vi "QuP Multiplexer Control.vi"() -> ()   [LabVIEW 2020, in "QuPMXdriver.lvlib"]
uses:
  QuPMXdriver.lvlib
  91754cce-ab52-4237-b78a-64c01c446f44.vi
  32ad12f4-2c8c-4504-800a-0d774754ae80.vi
  bf4f7028-8ca7-4759-aadb-7144e2be3c91.vi
  040f1b57-66c1-4072-aa26-6ea72dd8171f.vi
  6aed5eb3-691d-4dc6-b830-00691c629857.vi
  Sequence Editor.vi
  <vilib>/Comparison/Equal/Equal Functor/Equal Functor.lvclass
  cf69aa09-ab28-4be9-8615-1d2717454787.vi
panel:
  out "dummy for event \"check channels\"":bool
  in  "Set to sequence line:":i32=2 min=1 step=1
  in  "set sq line":bool
  out "Connected\nboards":bool[](array[boolean])
  in  "Get sq from MX":bool
  in  "Load sq to MX":bool
  in  "no sequences get":bool
  out "Number of sequence lines:":i32 min=0 step=1
  in  "sequence editor":bool
  out "Guards ref array":refnum<vi>[][](array[refnum])
  in  "G5C1":bool
  in  "G5C2":bool
  in  "G6C1":bool
  in  "G6C2":bool
  in  "G4C1":bool
  in  "G4C2":bool
  in  "G3C1":bool
  in  "G3C2":bool
  in  "G2C1":bool
  in  "G2C2":bool
  in  "G1C1":bool
  in  "G1C2":bool
  out "No. of connected slave boards:":u32
  out "Slaves ref array":refnum<vi>[][](array[refnum])
  in  "S5C1":bool
  in  "S5C2":bool
  in  "S6C1":bool
  in  "S6C2":bool
  in  "S4C1":bool
  in  "S4C2":bool
  in  "S3C1":bool
  in  "S3C2":bool
  in  "S2C1":bool
  in  "S2C2":bool
  in  "S1C1":bool
  in  "S1C2":bool
  in  "init":bool
  in  "Get Status":bool
  out "Ready?":bool=TRUE
  out "Enabled":bool=TRUE
  in  "check channels":bool
  in  "delay get":bool
  in  "delay set":bool
  in  "Enable\nDelay (ms)":dbl=2.0 min=0.8
  in  "timer get":bool
  in  "timer set":bool
  in  "Timer (ms)":i32=1000 min=0 step=1
  in  "Trigger polarity":enum32{"Positive", "Negative"}(radio)
  in  "Trigger source":enum32{"Internal", "External"}(radio)
  out "FP":refnum<vi>[](array[refnum])
  in  "Operation":enum32{"Remote", "Local"}(radio)=enum."Local"
  out "ID":string
  in  "reset":bool
  in  "clear":bool
  in  "stop":bool
  in  "start":bool
  in  "resume":bool
  in  "pause":bool
  in  "Stop":bool
  out "error":errorcluster
  in  "VISA":refnum<visa-resource-name>
  # "Channels"
  # "Properties"
  # "Slave boards"
  # "1       2      3      4      5      6"
  # "Channel 1"
  # "Channel 2"
  # "1       2      3      4      5      6"
  # "Guards"
  # "Channel 1"
  # "These are buttons,\nclick it!"
  # "Channel 2"
  # "Sequence"
  # "Error"
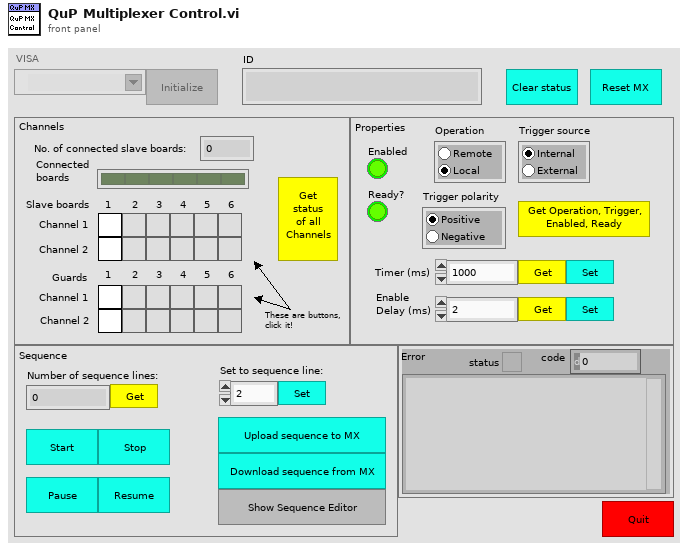
[diagram p1: front panel]
types:
  T1 = enum8{"Enabled", "Disabled", "Disabled and Grayed Out"}
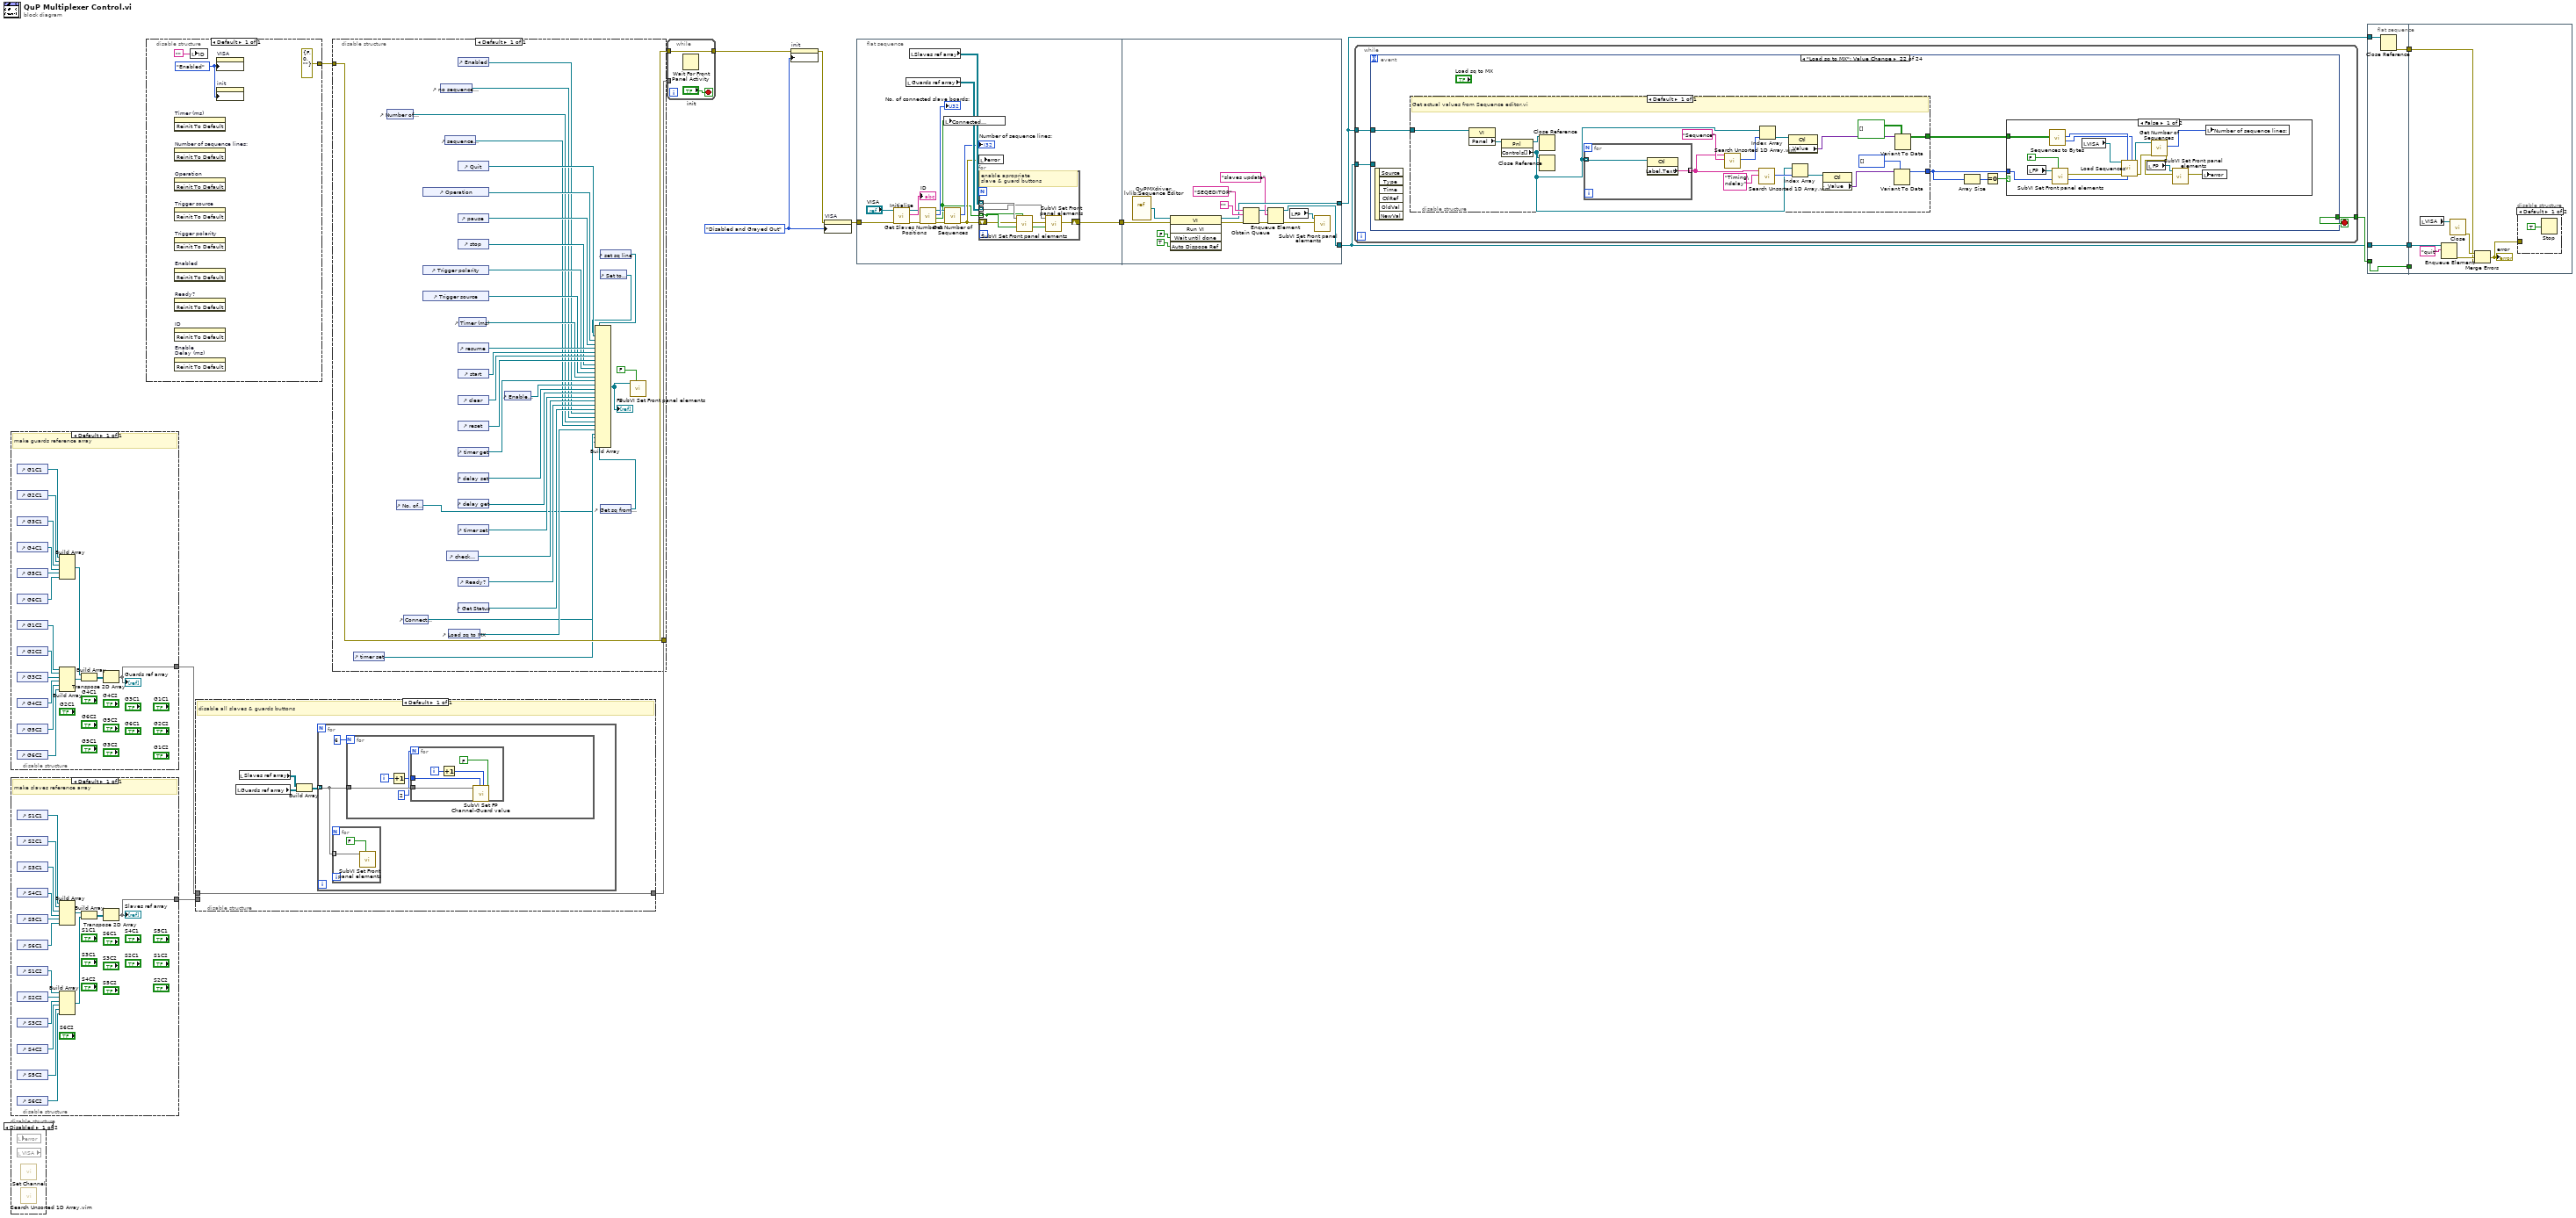
[diagram p0: block diagram]
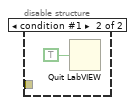
[diagram p3: hidden frame]
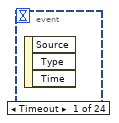
[diagram p4: hidden frame]
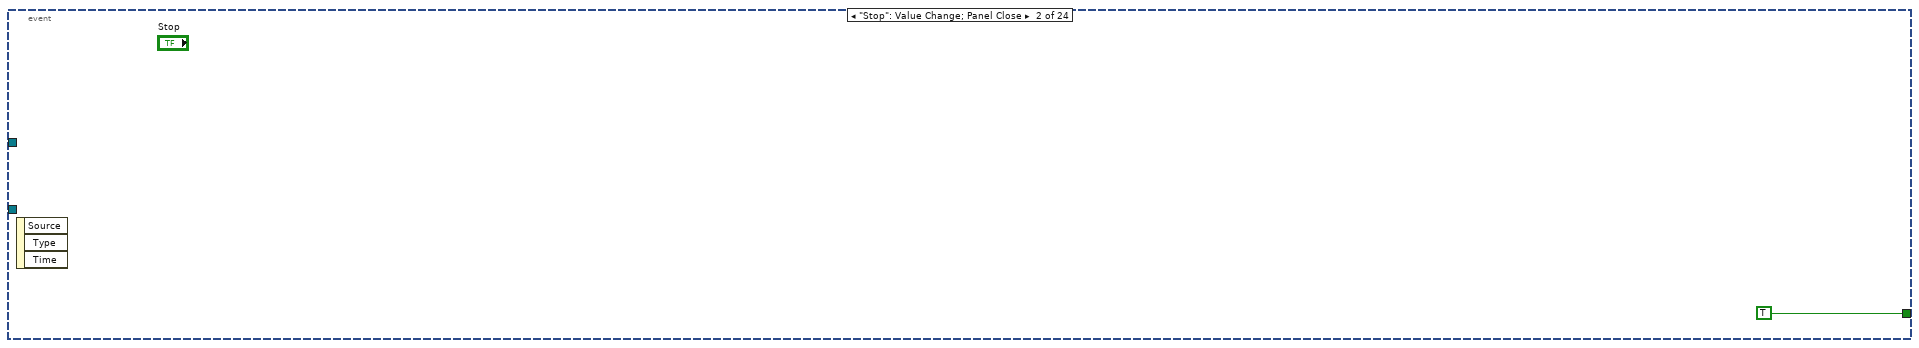
[diagram p5: hidden frame]
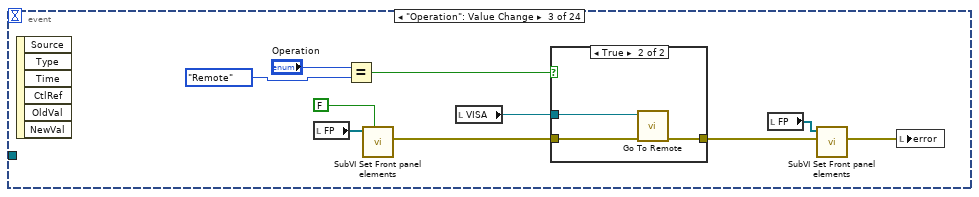
[diagram p6: hidden frame]
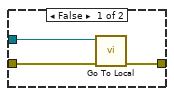
[diagram p7: hidden frame]
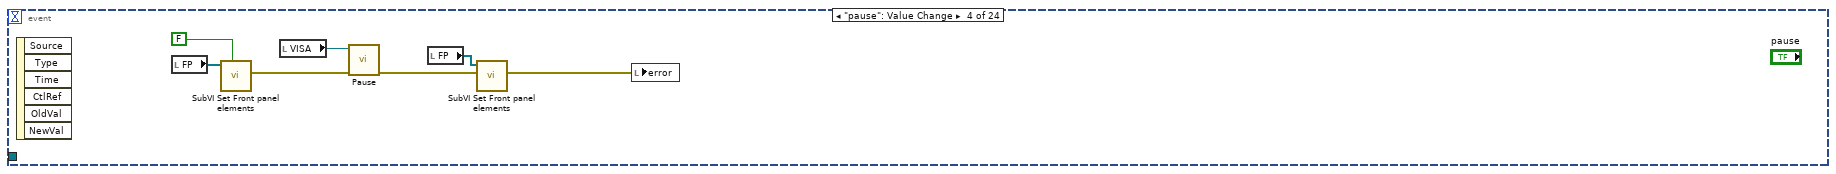
[diagram p8: hidden frame]
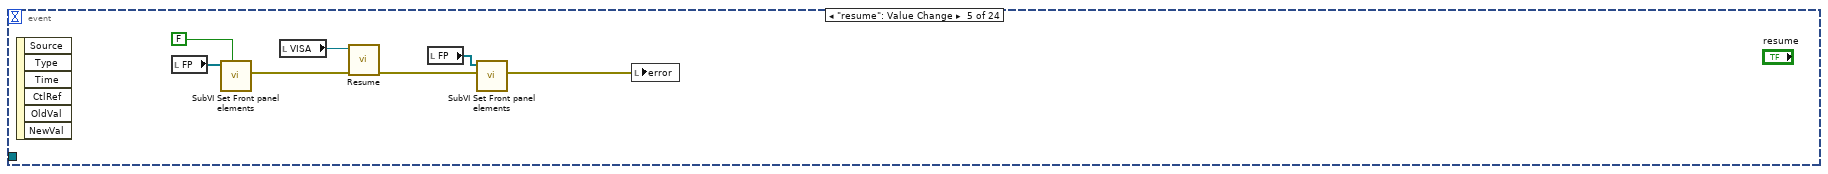
[diagram p9: hidden frame]
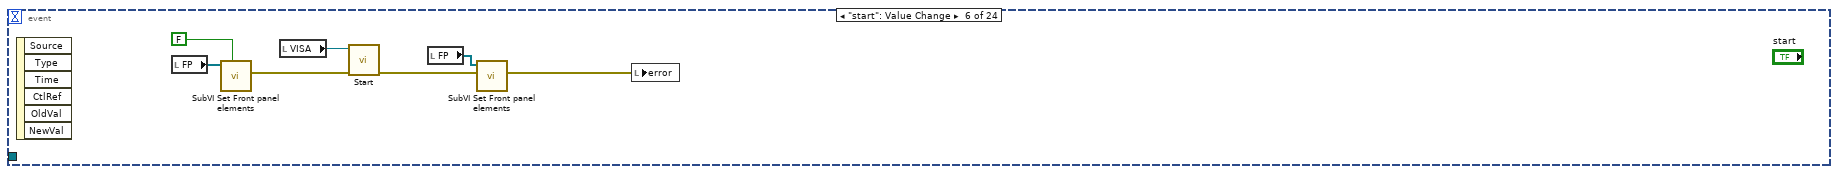
[diagram p10: hidden frame]
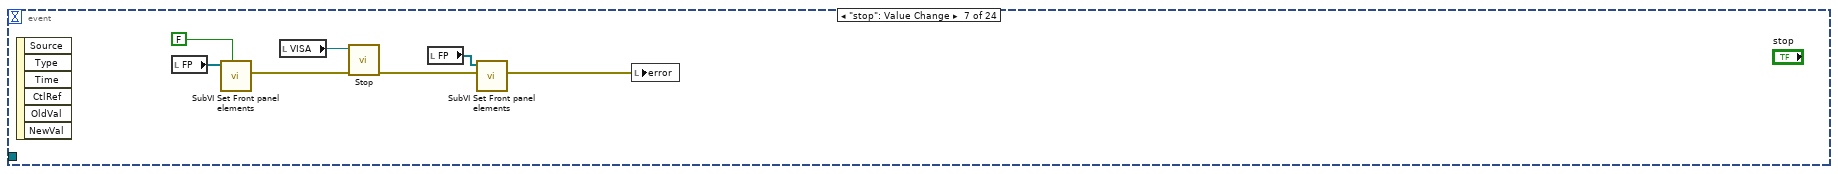
[diagram p11: hidden frame]
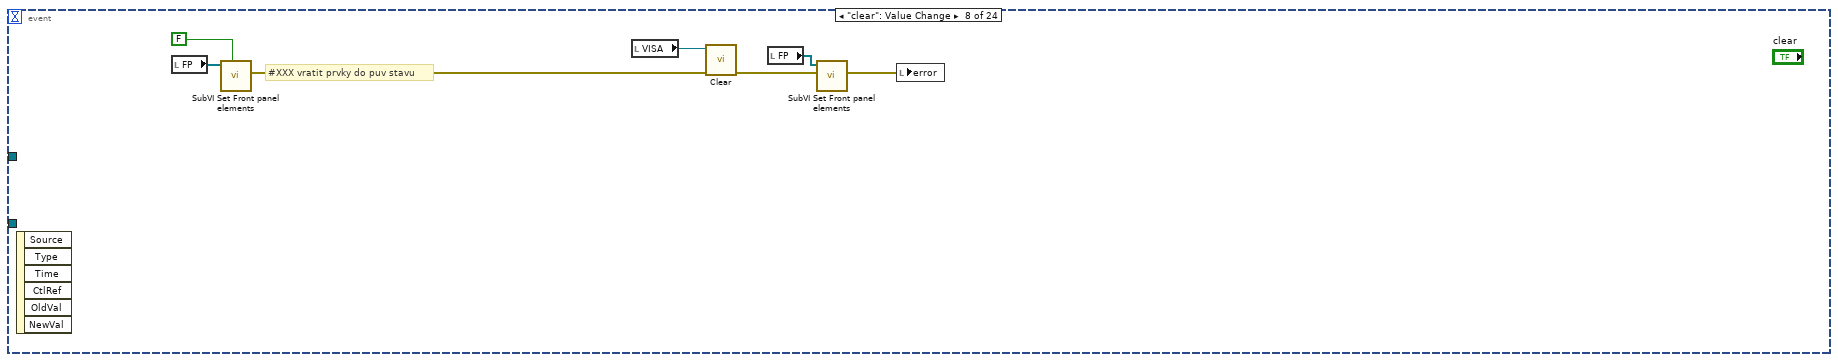
[diagram p12: hidden frame]
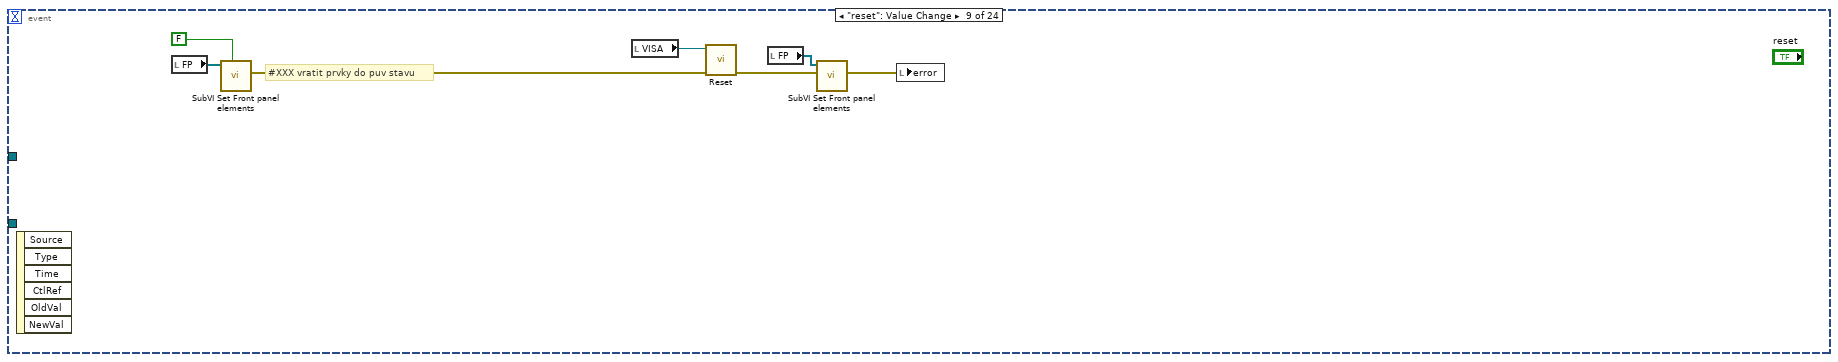
[diagram p13: hidden frame]
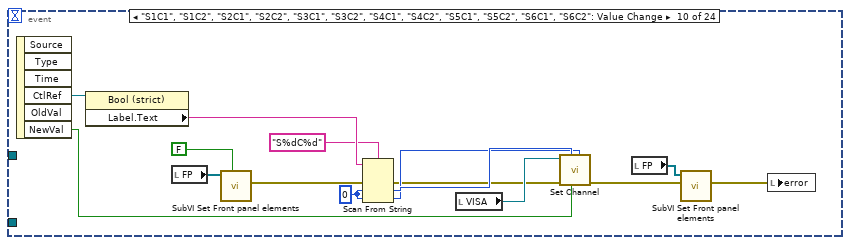
[diagram p14: hidden frame]
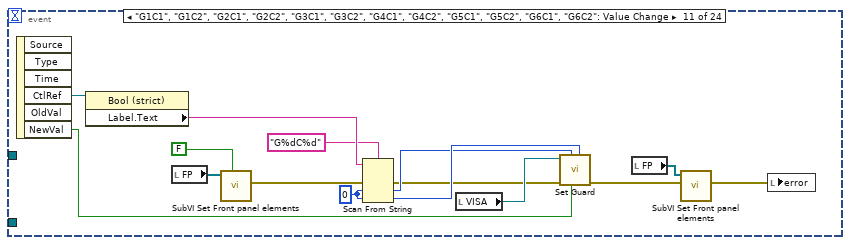
[diagram p15: hidden frame]
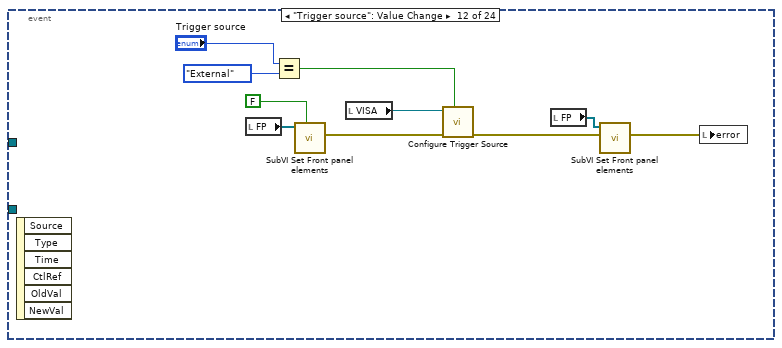
[diagram p16: hidden frame]
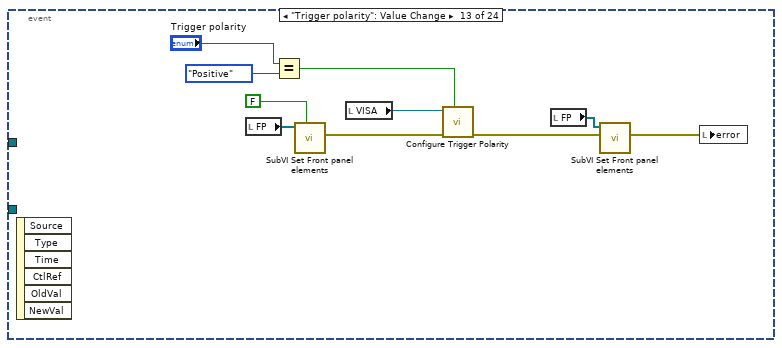
[diagram p17: hidden frame]
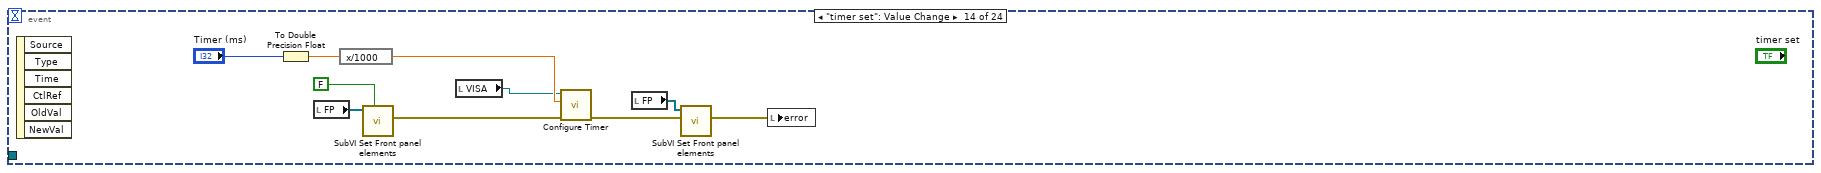
[diagram p18: hidden frame]
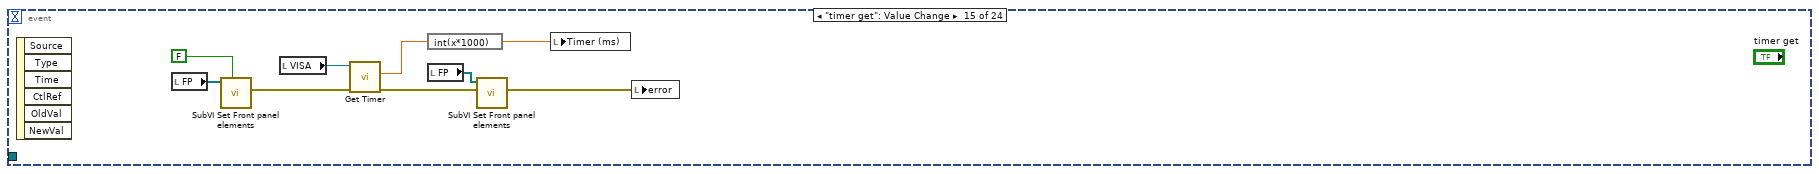
[diagram p19: hidden frame]
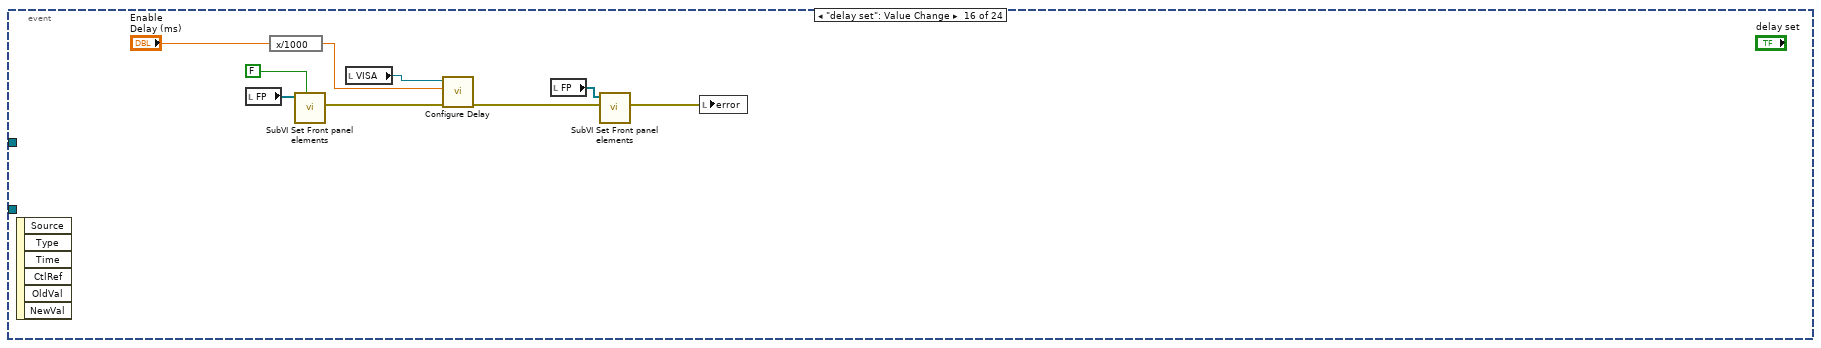
[diagram p20: hidden frame]
diagram:
  w12 = T1."Disabled and Grayed Out" ("Disabled")
  n1 = disable-structure shown="Default" {
    disable-tunnel: [w17] -> w9
    frame Enabled {
      # "make guards reference array"
      n2 = control-ref of="G1C1"() -> (w25:refnum<vi>)
      n3 = control-ref of="G2C1"() -> (w26:refnum<vi>)
      n4 = control-ref of="G3C1"() -> (w27:refnum<vi>)
      n5 = control-ref of="G4C1"() -> (w28:refnum<vi>)
      n6 = control-ref of="G5C1"() -> (w29:refnum<vi>)
      n7 = control-ref of="G6C1"() -> (w30:refnum<vi>)
      n8 = control-ref of="G1C2"() -> (w18:refnum<vi>)
      n9 = control-ref of="G2C2"() -> (w19:refnum<vi>)
      n10 = control-ref of="G3C2"() -> (w20:refnum<vi>)
      n11 = control-ref of="G4C2"() -> (w21:refnum<vi>)
      n12 = control-ref of="G5C2"() -> (w22:refnum<vi>)
      n13 = control-ref of="G6C2"() -> (w23:refnum<vi>)
      n14 = Build Array(w25, w26, w27, w28, w29, w30) -> (w24:refnum<vi>[])
      n15 = Build Array(w18, w19, w20, w21, w22, w23) -> (w31:refnum<vi>[])
      n16 = Build Array(w24, w31) -> (w32:refnum<vi>[][])
      n17 = Transpose 2D Array(2D array=w32) -> (transposed array=w17:refnum<vi>[][])
      "Guards ref array" <- w17
    }
  }
  n18 = disable-structure shown="Default" {
    disable-tunnel: [w33] -> w10
    frame Enabled {
      # "make slaves reference array"
      n19 = control-ref of="S1C1"() -> (w48:refnum<vi>)
      n20 = control-ref of="S2C1"() -> (w47:refnum<vi>)
      n21 = control-ref of="S3C1"() -> (w46:refnum<vi>)
      n22 = control-ref of="S4C1"() -> (w45:refnum<vi>)
      n23 = control-ref of="S5C1"() -> (w44:refnum<vi>)
      n24 = control-ref of="S6C1"() -> (w43:refnum<vi>)
      n25 = control-ref of="S1C2"() -> (w42:refnum<vi>)
      n26 = control-ref of="S2C2"() -> (w41:refnum<vi>)
      n27 = control-ref of="S3C2"() -> (w40:refnum<vi>)
      n28 = control-ref of="S4C2"() -> (w39:refnum<vi>)
      n29 = control-ref of="S5C2"() -> (w38:refnum<vi>)
      n30 = control-ref of="S6C2"() -> (w37:refnum<vi>)
      n31 = Build Array(w48, w47, w46, w45, w44, w43) -> (w35:refnum<vi>[])
      n32 = Build Array(w42, w41, w40, w39, w38, w37) -> (w36:refnum<vi>[])
      n33 = Build Array(w35, w36) -> (w34:refnum<vi>[][])
      n34 = Transpose 2D Array(2D array=w34) -> (transposed array=w33:refnum<vi>[][])
      "Slaves ref array" <- w33
    }
  }
  n35 = disable-structure shown="Disabled" {
    frame Disabled {
      n36 = local read "error"() -> ()  [unwired: 1 in]
      n37 = local read "VISA"() -> ()  [unwired: 1 out]
      n38 = call "Set Channel.vi"() -> ()  [unwired: 10 in, 2 out]
      n39 = call "Search Unsorted 1D Array.vim"() -> ()  [unwired: 11 in, 1 out]
    }
    frame Enabled {
    }
  }
  n40 = disable-structure shown="Default" {
    disable-tunnel: [errorcluster {"status"=FALSE, "code"=0, "source"=""} ("error in (no error)")] -> w2
    frame Enabled {
      w51 = T1."Enabled" ("Disabled")
      n41 = invoke on="Timer (ms)" class="DigNum (strict)" method="Reinit To Default"() -> ()  [unwired: 3 in, 3 out]
      n42 = invoke on="Number of sequence lines:" class="DigNum (strict)" method="Reinit To Default"() -> ()  [unwired: 3 in, 3 out]
      n43 = invoke on="Operation" class="RadioBtnsControl (strict)" method="Reinit To Default"() -> ()  [unwired: 3 in, 3 out]
      n44 = invoke on="Trigger source" class="RadioBtnsControl (strict)" method="Reinit To Default"() -> ()  [unwired: 3 in, 3 out]
      n45 = invoke on="Trigger polarity" class="RadioBtnsControl (strict)" method="Reinit To Default"() -> ()  [unwired: 3 in, 3 out]
      n46 = invoke on="Enabled" class="Bool (strict)" method="Reinit To Default"() -> ()  [unwired: 3 in, 3 out]
      n47 = invoke on="Ready?" class="Bool (strict)" method="Reinit To Default"() -> ()  [unwired: 3 in, 3 out]
      n48 = invoke on="ID" class="Str" method="Reinit To Default"() -> ()  [unwired: 3 in, 3 out]
      n49 = invoke on="Enable\nDelay (ms)" class="DigNum (strict)" method="Reinit To Default"() -> ()  [unwired: 3 in, 3 out]
      n50 = local write "ID"("") -> ()
      n51 = property on="VISA" class="VISAName"("DisabledEnum"=w51) -> ()  [unwired: 2 in, 2 out]
      n52 = property on="init" class="Bool"("DisabledEnum"=w51) -> ()  [unwired: 2 in, 2 out]
    }
  }
  n53 = disable-structure shown="Default" {
    disable-tunnel: w10 -> [_]
    disable-tunnel: w9 -> [w52]
    disable-tunnel: [w52] -> w8
    frame Enabled {
      # "disable all slaves & guards buttons"
      n54 = local read "Guards ref array"() -> (w53:refnum<vi>[][])
      n55 = local read "Slaves ref array"() -> (w55:refnum<vi>[][])
      n56 = Build Array(w55, w53) -> (w54:refnum<vi>[][][])
      n57 = for {
        tunnel: w54 -> [w56] mode=indexing
        n58 = for {
          tunnel: w56 -> [w68] mode=indexing
          n59 = call "SubVI Set Front panel elements.vi"("Enable elements (T)"=FALSE, "Array"=w68) -> ()  [unwired: 9 in, 1 out]
        }
        n60 = for {
          N: 6 -> [_]
          tunnel: w56 -> [w61]
          i -> [w59]
          n61 = Increment(x=w59) -> (x+1=w58:i32)
          n62 = for {
            N: 2 -> [_]
            tunnel: w61 -> [w66]
            tunnel: w58 -> [w64]
            i -> [w63]
            n63 = Increment(x=w63) -> (x+1=w62:i32)
            n64 = call "SubVI Set FP Channel-Guard value.vi"("Value"=FALSE, "Ch ID"=w62, "Slave ID"=w64, "Slaves ref array"=w66) -> ()  [unwired: 7 in, 1 out]
          }
        }
      }
    }
  }
  n65 = disable-structure shown="Default" {
    disable-tunnel: [w75] -> w1
    disable-tunnel: w2 -> [w75]
    frame Enabled {
      n66 = control-ref of="timer set"() -> (w74:refnum<vi>)
      n67 = control-ref of="Number of sequence lines:"() -> (w78:refnum<vi>)
      n68 = control-ref of="No. of connected slave boards:"() -> (w72:refnum<vi>)
      n69 = control-ref of="Connected\nboards"() -> (w73:refnum<vi>)
      n70 = control-ref of="Operation"() -> (w100:refnum<vi>)
      n71 = control-ref of="Trigger polarity"() -> (w91:refnum<vi>)
      n72 = control-ref of="Trigger source"() -> (w90:refnum<vi>)
      n73 = control-ref of="no sequences get"() -> (w79:refnum<vi>)
      n74 = control-ref of="sequence editor"() -> (w77:refnum<vi>)
      n75 = control-ref of="check channels"() -> (w83:refnum<vi>)
      n76 = control-ref of="Load sq to MX"() -> (w76:refnum<vi>)
      n77 = control-ref of="Enabled"() -> (w80:refnum<vi>)
      n78 = control-ref of="Quit"() -> (w101:refnum<vi>)
      n79 = control-ref of="pause"() -> (w99:refnum<vi>)
      n80 = control-ref of="stop"() -> (w92:refnum<vi>)
      n81 = control-ref of="resume"() -> (w98:refnum<vi>)
      n82 = control-ref of="start"() -> (w97:refnum<vi>)
      n83 = control-ref of="clear"() -> (w96:refnum<vi>)
      n84 = control-ref of="reset"() -> (w95:refnum<vi>)
      n85 = control-ref of="timer get"() -> (w88:refnum<vi>)
      n86 = control-ref of="delay set"() -> (w86:refnum<vi>)
      n87 = control-ref of="delay get"() -> (w85:refnum<vi>)
      n88 = control-ref of="timer set"() -> (w84:refnum<vi>)
      n89 = control-ref of="Ready?"() -> (w82:refnum<vi>)
      n90 = control-ref of="Get Status"() -> (w81:refnum<vi>)
      n91 = control-ref of="Timer (ms)"() -> (w89:refnum<vi>)
      n92 = control-ref of="Enable\nDelay (ms)"() -> (w87:refnum<vi>)
      n93 = control-ref of="set sq line"() -> (w69:refnum<vi>)
      n94 = control-ref of="Set to sequence line:"() -> (w70:refnum<vi>)
      n95 = control-ref of="Get sq from MX"() -> (w71:refnum<vi>)
      n96 = Build Array(w69, w70, w101, w100, w99, w98, w97, w96, w95, w92, w91, w90, w89, w88, w87, w86, w85, w84, w83, w82, w81, w80, w79, w78, w77, w76, w74, w73, w72, w71) -> (w94:refnum<vi>[])
      "FP" <- w94
      n97 = call "SubVI Set Front panel elements.vi"("Enable elements (T)"=FALSE ("Enable elements"), "Array"=w94) -> ()  [unwired: 9 in, 1 out]
    }
  }
  n98 = while {
    tunnel: [w102] -> w15
    tunnel: w8 -> [_]
    tunnel: w1 -> [w102]
    stop <- "init" stop-if-true
    n99 = Wait For Front Panel Activity() -> ()  [unwired: 3 in, 1 out]
  }
  n100 = property on="init" class="Bool"(error in=w15, "DisabledEnum"=w12) -> (error out=w14:errorcluster)  [unwired: 1 in, 1 out]
  n101 = property on="VISA" class="VISAName"(error in=w14, "DisabledEnum"=w12) -> (error out=w13:errorcluster)  [unwired: 1 in, 1 out]
  n102 = flat-sequence {
    tunnel: w13 -> [w117]
    tunnel: [w110] -> w11
    tunnel: w11 -> [w128]
    tunnel: [w124] -> w7
    tunnel: [w131] -> w3
    frame #0 {
      n103 = call "Initialize.vi"("error in (no error)"=w117, "VISA resource name"="VISA") -> ("error out"=w115:errorcluster, "ID"=→"ID":string, "VISA resource name out"=w114:refnum<visa-resource-name>)  [unwired: 7 in]
      n104 = local read "Guards ref array"() -> (w111:refnum<vi>[][])
      n105 = local read "Slaves ref array"() -> (w112:refnum<vi>[][])
      n106 = call "Get Slaves Number & Positions.vi"("error in (no error)"=w115, "VISA resource name"=w114) -> ("error out"=w109:errorcluster, "Connected Slaves"=w104:bool[], "No. of Slaves"=→"No. of connected slave boards:":u32, "VISA resource name out"=w107:refnum<visa-resource-name>)  [unwired: 6 in]
      n107 = local write "Connected\nboards"(w104) -> ()
      n108 = call "Get Number of Sequences.vi"("error in (no error)"=w109, "VISA resource name"=w107) -> ("error out"=w108:errorcluster, "Number of sequences"=→"Number of sequence lines:":i32)  [unwired: 7 in, 1 out]
      n109 = local write "error"(w108) -> ()
      n110 = for {
        tunnel: w112 -> [w123] mode=indexing
        tunnel: w104 -> [w121] mode=indexing
        tunnel: w111 -> [w122] mode=indexing
        shift-right: [w119] -> w110
        shift-left: w108 -> [w118]
        # "enable apropriate\nslave & guard buttons"
        n111 = call "SubVI Set Front panel elements.vi"("Enable elements (T)"=w121, "error in (passthrough)"=w118, "Array"=w123) -> ("error out"=w120:errorcluster)  [unwired: 8 in]
        n112 = call "SubVI Set Front panel elements.vi"("Enable elements (T)"=w121, "error in (passthrough)"=w120, "Array"=w122) -> ("error out"=w119:errorcluster)  [unwired: 8 in]
      }
    }
    frame #1 {
      n113 = vi-ref "QuPMXdriver.lvlib:Sequence Editor.vi"() -> (w136:refnum<vi>)
      n114 = invoke class="VI" method="Run VI"(reference=w136, error in=w128, "Wait until done"=FALSE ("Wait Until Done"), "Auto Dispose Ref"=TRUE ("Wait Until Done")) -> (reference out=w131:refnum<vi>, error out=w132:errorcluster)  [unwired: 1 in, 3 out]
      n115 = Obtain Queue(name (unnamed)="SEQEDITOR", element data type="", error in (no error)=w132) -> (queue out=w125:refnum<queue>, error out=w127:errorcluster)  [unwired: 2 in, 1 out]
      n116 = Enqueue Element(queue=w125, element="slaves update", error in (no error)=w127) -> (queue out=w124:refnum<queue>, error out=w126:errorcluster)  [unwired: 1 in, 1 out]
      n117 = local read "FP"() -> (w137:refnum<vi>[])
      n118 = call "SubVI Set Front panel elements.vi"("error in (passthrough)"=w126, "Array"=w137) -> ()  [unwired: 9 in, 1 out]
    }
  }
  n119 = while {
    tunnel: [w140] -> w16
    tunnel: w7 -> [w139]
    tunnel: w3 -> [w138]
    stop <- w140 stop-if-true
    n120 = event shown="[21] \"Load sq to MX\": Value Change" {
      selector: _ -> [_ _ _ _ _ _ _ _ _ _ _ _ _ _ _ _ _ _ _ _ _ _ _ _]
      dyn-events: _ -> [_ _ _ _ _ _ _ _ _ _ _ _ _ _ _ _ _ _ _ _ _ _ _ _]
      timeout: _ -> [_ _ _ _ _ _ _ _ _ _ _ _ _ _ _ _ _ _ _ _ _ _ _ _]
      tunnel: [_ TRUE ("Stop") _ _ _ _ _ _ _ _ _ _ _ _ _ _ _ _ _ _ _ _ _ _] -> w140
      tunnel: w139 -> [_ _ _ _ _ _ _ _ _ _ _ _ _ _ _ _ _ w289 _ _ w353 _ _ w430]
      tunnel: w138 -> [_ _ _ _ _ _ _ _ _ _ _ _ _ _ _ _ _ _ _ _ _ w358 w406 w433]
      event Timeout {
        n121 = event-data() -> ()  [unwired: 1 in, 3 out]
      }
      event "Stop": Value Change; Panel Close {
        n122 = event-data() -> ()  [unwired: 1 in, 3 out]
      }
      event "Operation": Value Change {
        n123 = event-data() -> ()  [unwired: 1 in, 6 out]
        n124 = local read "FP"() -> (w147:refnum<vi>[])
        n125 = Equal?(x="Operation", y=enum32{"Remote", "Local"}."Remote") -> (x = y?=w148:bool)
        n126 = call "SubVI Set Front panel elements.vi"("Enable elements (T)"=FALSE, "Array"=w147) -> ("error out"=w145:errorcluster)  [unwired: 9 in]
        n127 = local read "VISA"() -> (w151:refnum<visa-resource-name>)
        n128 = case shown="True" w148 {
          tunnel: [w154 w157] -> w144
          tunnel: w151 -> [w153 w156]
          tunnel: w145 -> [w152 w155]
          frame False {
            n129 = call "Go To Local.vi"("error in (no error)"=w152, "VISA resource name"=w153) -> ("error out"=w154:errorcluster)  [unwired: 8 in, 1 out]
          }
          frame True {
            n130 = call "Go To Remote.vi"("error in (no error)"=w155, "VISA resource name"=w156) -> ("error out"=w157:errorcluster)  [unwired: 8 in, 1 out]
          }
        }
        n131 = local read "FP"() -> (w142:refnum<vi>[])
        n132 = call "SubVI Set Front panel elements.vi"("error in (passthrough)"=w144, "Array"=w142) -> ("error out"=w143:errorcluster)  [unwired: 9 in]
        n133 = local write "error"(w143) -> ()
      }
      event "pause": Value Change {
        n134 = event-data() -> ()  [unwired: 1 in, 6 out]
        n135 = local read "FP"() -> (w163:refnum<vi>[])
        n136 = call "SubVI Set Front panel elements.vi"("Enable elements (T)"=FALSE, "Array"=w163) -> ("error out"=w160:errorcluster)  [unwired: 9 in]
        n137 = local read "VISA"() -> (w164:refnum<visa-resource-name>)
        n138 = call "Pause.vi"("error in (no error)"=w160, "VISA resource name"=w164) -> ("error out"=w159:errorcluster)  [unwired: 8 in, 1 out]
        n139 = local read "FP"() -> (w161:refnum<vi>[])
        n140 = call "SubVI Set Front panel elements.vi"("error in (passthrough)"=w159, "Array"=w161) -> ("error out"=w158:errorcluster)  [unwired: 9 in]
        n141 = local write "error"(w158) -> ()
      }
      event "resume": Value Change {
        n142 = event-data() -> ()  [unwired: 1 in, 6 out]
        n143 = local read "FP"() -> (w169:refnum<vi>[])
        n144 = call "SubVI Set Front panel elements.vi"("Enable elements (T)"=FALSE, "Array"=w169) -> ("error out"=w167:errorcluster)  [unwired: 9 in]
        n145 = local read "VISA"() -> (w171:refnum<visa-resource-name>)
        n146 = call "Resume.vi"("error in (no error)"=w167, "VISA resource name"=w171) -> ("error out"=w166:errorcluster)  [unwired: 8 in, 1 out]
        n147 = local read "FP"() -> (w170:refnum<vi>[])
        n148 = call "SubVI Set Front panel elements.vi"("error in (passthrough)"=w166, "Array"=w170) -> ("error out"=w165:errorcluster)  [unwired: 9 in]
        n149 = local write "error"(w165) -> ()
      }
      event "start": Value Change {
        n150 = event-data() -> ()  [unwired: 1 in, 6 out]
        n151 = local read "FP"() -> (w176:refnum<vi>[])
        n152 = call "SubVI Set Front panel elements.vi"("Enable elements (T)"=FALSE, "Array"=w176) -> ("error out"=w174:errorcluster)  [unwired: 9 in]
        n153 = local read "VISA"() -> (w178:refnum<visa-resource-name>)
        n154 = call "Start.vi"("error in (no error)"=w174, "VISA resource name"=w178) -> ("error out"=w173:errorcluster)  [unwired: 8 in, 1 out]
        n155 = local read "FP"() -> (w177:refnum<vi>[])
        n156 = call "SubVI Set Front panel elements.vi"("error in (passthrough)"=w173, "Array"=w177) -> ("error out"=w172:errorcluster)  [unwired: 9 in]
        n157 = local write "error"(w172) -> ()
      }
      event "stop": Value Change {
        n158 = event-data() -> ()  [unwired: 1 in, 6 out]
        n159 = local read "FP"() -> (w183:refnum<vi>[])
        n160 = call "SubVI Set Front panel elements.vi"("Enable elements (T)"=FALSE, "Array"=w183) -> ("error out"=w181:errorcluster)  [unwired: 9 in]
        n161 = local read "VISA"() -> (w185:refnum<visa-resource-name>)
        n162 = call "Stop.vi"("error in (no error)"=w181, "VISA resource name"=w185) -> ("error out"=w180:errorcluster)  [unwired: 8 in, 1 out]
        n163 = local read "FP"() -> (w184:refnum<vi>[])
        n164 = call "SubVI Set Front panel elements.vi"("error in (passthrough)"=w180, "Array"=w184) -> ("error out"=w179:errorcluster)  [unwired: 9 in]
        n165 = local write "error"(w179) -> ()
      }
      event "clear": Value Change {
        # "#XXX vratit prvky do puv stavu"
        n166 = event-data() -> ()  [unwired: 1 in, 6 out]
        n167 = local read "FP"() -> (w190:refnum<vi>[])
        n168 = call "SubVI Set Front panel elements.vi"("Enable elements (T)"=FALSE, "Array"=w190) -> ("error out"=w188:errorcluster)  [unwired: 9 in]
        n169 = local read "VISA"() -> (w192:refnum<visa-resource-name>)
        n170 = call "Clear.vi"("error in (no error)"=w188, "VISA resource name"=w192) -> ("error out"=w187:errorcluster)  [unwired: 8 in, 1 out]
        n171 = local read "FP"() -> (w191:refnum<vi>[])
        n172 = call "SubVI Set Front panel elements.vi"("error in (passthrough)"=w187, "Array"=w191) -> ("error out"=w186:errorcluster)  [unwired: 9 in]
        n173 = local write "error"(w186) -> ()
      }
      event "reset": Value Change {
        # "#XXX vratit prvky do puv stavu"
        n174 = event-data() -> ()  [unwired: 1 in, 6 out]
        n175 = local read "FP"() -> (w197:refnum<vi>[])
        n176 = call "SubVI Set Front panel elements.vi"("Enable elements (T)"=FALSE, "Array"=w197) -> ("error out"=w195:errorcluster)  [unwired: 9 in]
        n177 = local read "VISA"() -> (w199:refnum<visa-resource-name>)
        n178 = call "Reset.vi"("error in (no error)"=w195, "VISA resource name"=w199) -> ("error out"=w194:errorcluster)  [unwired: 8 in, 1 out]
        n179 = local read "FP"() -> (w198:refnum<vi>[])
        n180 = call "SubVI Set Front panel elements.vi"("error in (passthrough)"=w194, "Array"=w198) -> ("error out"=w193:errorcluster)  [unwired: 9 in]
        n181 = local write "error"(w193) -> ()
      }
      event "S1C1", "S1C2", "S2C1", "S2C2", "S3C1", "S3C2", "S4C1", "S4C2", "S5C1", "S5C2", "S6C1", "S6C2": Value Change {
        w200 = 0 ("default value 1")
        n182 = event-data() -> ("CtlRef"=w214:refnum<vi>, "NewVal"=w208:bool)  [unwired: 1 in, 4 out]
        n183 = property class="Bool (strict)"(reference=w214) -> ("Label.Text"=w213:string)  [unwired: 1 in, 2 out]
        n184 = local read "FP"() -> (w203:refnum<vi>[])
        n185 = call "SubVI Set Front panel elements.vi"("Enable elements (T)"=FALSE, "Array"=w203) -> ("error out"=w201:errorcluster)  [unwired: 9 in]
        n186 = Scan From String(format string="S%dC%d", input string=w213, error in=w201, default 1=w200, default 2=w200) -> (error out=w207:errorcluster, output 1=w211:i32, output 2=w210:i32)  [unwired: 1 in, 2 out]
        n187 = local read "VISA"() -> (w209:refnum<visa-resource-name>)
        n188 = call "Set Channel.vi"("Channel"=w210, "Channel Status"=w208, "Slave"=w211, "error in (no error)"=w207, "VISA resource name"=w209) -> ("error out"=w205:errorcluster)  [unwired: 5 in, 1 out]
        n189 = local read "FP"() -> (w206:refnum<vi>[])
        n190 = call "SubVI Set Front panel elements.vi"("error in (passthrough)"=w205, "Array"=w206) -> ("error out"=w204:errorcluster)  [unwired: 9 in]
        n191 = local write "error"(w204) -> ()
      }
      event "G1C1", "G1C2", "G2C1", "G2C2", "G3C1", "G3C2", "G4C1", "G4C2", "G5C1", "G5C2", "G6C1", "G6C2": Value Change {
        w221 = 0 ("default value 1")
        n192 = event-data() -> ("CtlRef"=w227:refnum<vi>, "NewVal"=w223:bool)  [unwired: 1 in, 4 out]
        n193 = property class="Bool (strict)"(reference=w227) -> ("Label.Text"=w229:string)  [unwired: 1 in, 2 out]
        n194 = local read "FP"() -> (w220:refnum<vi>[])
        n195 = call "SubVI Set Front panel elements.vi"("Enable elements (T)"=FALSE, "Array"=w220) -> ("error out"=w218:errorcluster)  [unwired: 9 in]
        n196 = Scan From String(format string="G%dC%d", input string=w229, error in=w218, default 1=w221, default 2=w221) -> (error out=w222:errorcluster, output 1=w225:i32, output 2=w226:i32)  [unwired: 1 in, 2 out]
        n197 = local read "VISA"() -> (w224:refnum<visa-resource-name>)
        n198 = call "Set Guard.vi"("Channel"=w226, "Channel Guard Status"=w223, "Slave"=w225, "error in (no error)"=w222, "VISA resource name"=w224) -> ("error out"=w216:errorcluster)  [unwired: 5 in, 1 out]
        n199 = local read "FP"() -> (w217:refnum<vi>[])
        n200 = call "SubVI Set Front panel elements.vi"("error in (passthrough)"=w216, "Array"=w217) -> ("error out"=w215:errorcluster)  [unwired: 9 in]
        n201 = local write "error"(w215) -> ()
      }
      event "Trigger source": Value Change {
        n202 = event-data() -> ()  [unwired: 1 in, 6 out]
        n203 = local read "FP"() -> (w237:refnum<vi>[])
        n204 = Equal?(x="Trigger source", y=enum32{"Internal", "External"}."External") -> (x = y?=w231:bool)
        n205 = call "SubVI Set Front panel elements.vi"("Enable elements (T)"=FALSE, "Array"=w237) -> ("error out"=w233:errorcluster)  [unwired: 9 in]
        n206 = local read "VISA"() -> (w235:refnum<visa-resource-name>)
        n207 = call "Configure Trigger Source.vi"("Trigger External (T)"=w231, "error in (no error)"=w233, "VISA resource name"=w235) -> ("error out"=w234:errorcluster)  [unwired: 7 in, 1 out]
        n208 = local read "FP"() -> (w238:refnum<vi>[])
        n209 = call "SubVI Set Front panel elements.vi"("error in (passthrough)"=w234, "Array"=w238) -> ("error out"=w239:errorcluster)  [unwired: 9 in]
        n210 = local write "error"(w239) -> ()
      }
      event "Trigger polarity": Value Change {
        n211 = event-data() -> ()  [unwired: 1 in, 6 out]
        n212 = local read "FP"() -> (w247:refnum<vi>[])
        n213 = Equal?(x="Trigger polarity", y=enum32{"Positive", "Negative"}."Positive") -> (x = y?=w241:bool)
        n214 = call "SubVI Set Front panel elements.vi"("Enable elements (T)"=FALSE, "Array"=w247) -> ("error out"=w245:errorcluster)  [unwired: 9 in]
        n215 = local read "VISA"() -> (w240:refnum<visa-resource-name>)
        n216 = call "Configure Trigger Polarity.vi"("Trigger Polarity Positive (T)"=w241, "error in (no error)"=w245, "VISA resource name"=w240) -> ("error out"=w244:errorcluster)  [unwired: 7 in, 1 out]
        n217 = local read "FP"() -> (w248:refnum<vi>[])
        n218 = call "SubVI Set Front panel elements.vi"("error in (passthrough)"=w244, "Array"=w248) -> ("error out"=w249:errorcluster)  [unwired: 9 in]
        n219 = local write "error"(w249) -> ()
      }
      event "timer set": Value Change {
        n220 = event-data() -> ()  [unwired: 1 in, 6 out]
        n221 = To Double Precision Float(number="Timer (ms)") -> (double precision float=w254:dbl)
        n222 = local read "FP"() -> (w257:refnum<vi>[])
        n223 = expression code="x/1000"(w254) -> (w253:dbl)
        n224 = call "SubVI Set Front panel elements.vi"("Enable elements (T)"=FALSE, "Array"=w257) -> ("error out"=w251:errorcluster)  [unwired: 9 in]
        n225 = local read "VISA"() -> (w252:refnum<visa-resource-name>)
        n226 = call "Configure Timer.vi"("error in (no error)"=w251, "Internal timer (2 s)"=w253, "VISA resource name"=w252) -> ("error out"=w250:errorcluster)  [unwired: 7 in, 1 out]
        n227 = local read "FP"() -> (w258:refnum<vi>[])
        n228 = call "SubVI Set Front panel elements.vi"("error in (passthrough)"=w250, "Array"=w258) -> ("error out"=w259:errorcluster)  [unwired: 9 in]
        n229 = local write "error"(w259) -> ()
      }
      event "timer get": Value Change {
        n230 = event-data() -> ()  [unwired: 1 in, 6 out]
        n231 = local read "FP"() -> (w266:refnum<vi>[])
        n232 = call "SubVI Set Front panel elements.vi"("Enable elements (T)"=FALSE, "Array"=w266) -> ("error out"=w264:errorcluster)  [unwired: 9 in]
        n233 = local read "VISA"() -> (w262:refnum<visa-resource-name>)
        n234 = call "Get Timer.vi"("error in (no error)"=w264, "VISA resource name"=w262) -> ("error out"=w263:errorcluster, "Internal Timer value (s)"=w261:dbl)  [unwired: 7 in, 1 out]
        n235 = expression code="int(x*1000)"(w261) -> (w260:dbl)
        n236 = local read "FP"() -> (w267:refnum<vi>[])
        n237 = call "SubVI Set Front panel elements.vi"("error in (passthrough)"=w263, "Array"=w267) -> ("error out"=w268:errorcluster)  [unwired: 9 in]
        n238 = local write "Timer (ms)"(w260) -> ()
        n239 = local write "error"(w268) -> ()
      }
      event "delay set": Value Change {
        n240 = event-data() -> ()  [unwired: 1 in, 6 out]
        n241 = local read "FP"() -> (w275:refnum<vi>[])
        n242 = expression code="x/1000"("Enable\nDelay (ms)") -> (w270:dbl)
        n243 = call "SubVI Set Front panel elements.vi"("Enable elements (T)"=FALSE, "Array"=w275) -> ("error out"=w272:errorcluster)  [unwired: 9 in]
        n244 = local read "VISA"() -> (w273:refnum<visa-resource-name>)
        n245 = call "Configure Delay.vi"("error in (no error)"=w272, "Delay (s)"=w270, "VISA resource name"=w273) -> ("error out"=w271:errorcluster)  [unwired: 7 in, 1 out]
        n246 = local read "FP"() -> (w276:refnum<vi>[])
        n247 = call "SubVI Set Front panel elements.vi"("error in (passthrough)"=w271, "Array"=w276) -> ("error out"=w277:errorcluster)  [unwired: 9 in]
        n248 = local write "error"(w277) -> ()
      }
      event "delay get": Value Change {
        n249 = event-data() -> ()  [unwired: 1 in, 6 out]
        n250 = local read "FP"() -> (w284:refnum<vi>[])
        n251 = call "SubVI Set Front panel elements.vi"("Enable elements (T)"=FALSE, "Array"=w284) -> ("error out"=w282:errorcluster)  [unwired: 9 in]
        n252 = local read "VISA"() -> (w280:refnum<visa-resource-name>)
        n253 = call "Get Delay.vi"("error in (no error)"=w282, "VISA resource name"=w280) -> ("error out"=w281:errorcluster, "Delay (s)"=w279:dbl)  [unwired: 7 in, 1 out]
        n254 = expression code="int(x*1000)"(w279) -> (w278:dbl)
        n255 = local read "FP"() -> (w285:refnum<vi>[])
        n256 = call "SubVI Set Front panel elements.vi"("error in (passthrough)"=w281, "Array"=w285) -> ("error out"=w286:errorcluster)  [unwired: 9 in]
        n257 = local write "Enable\nDelay (ms)"(w278) -> ()
        n258 = local write "error"(w286) -> ()
      }
      event "check channels", "dummy for event \"check channels\"": Value Change {
        # "this is only to get possibility\nto start this event case\neven if button \"check channels\"\nis latching"
        n259 = event-data() -> ()  [unwired: 1 in, 6 out]
        n260 = local read "FP"() -> (w301:refnum<vi>[])
        n261 = call "SubVI Set Front panel elements.vi"("Enable elements (T)"=FALSE, "Array"=w301) -> ("error out"=w294:errorcluster)  [unwired: 9 in]
        n262 = local read "VISA"() -> (w295:refnum<visa-resource-name>)
        n263 = local read "Guards ref array"() -> (w291:refnum<vi>[][])
        n264 = local read "Slaves ref array"() -> (w297:refnum<vi>[][])
        n265 = call "Get Slaves Number & Positions.vi"("error in (no error)"=w294, "VISA resource name"=w295) -> ("error out"=w292:errorcluster, "Connected Slaves"=w296:bool[], "No. of Slaves"=w298:u32)  [unwired: 6 in, 1 out]
        "Connected\nboards" <- w296
        n266 = local write "No. of connected slave boards:"(w298) -> ()
        n267 = for {
          tunnel: w297 -> [w309] mode=indexing
          tunnel: w296 -> [w305] mode=indexing
          shift-right: [w306] -> w293
          shift-left: w292 -> [w308]
          tunnel: w291 -> [w304] mode=indexing
          n268 = call "SubVI Set Front panel elements.vi"("Enable elements (T)"=w305, "error in (passthrough)"=w308, "Array"=w309) -> ("error out"=w307:errorcluster)  [unwired: 8 in]
          n269 = call "SubVI Set Front panel elements.vi"("Enable elements (T)"=w305, "error in (passthrough)"=w307, "Array"=w304) -> ("error out"=w306:errorcluster)  [unwired: 8 in]
        }
        n270 = for {
          N: 2 -> [_]
          shift-right: [w313] -> w288
          shift-left: w293 -> [w312]
          i -> [w311]
          n271 = Increment(x=w311) -> (x+1=w310:i32)
          n272 = for {
            N: 6 -> [_]
            shift-right: [w322] -> w313
            shift-left: w312 -> [w321]
            tunnel: w310 -> [w316]
            i -> [w319]
            # "#XXX no way how to check guard status?"
            n273 = local read "VISA"() -> (w320:refnum<visa-resource-name>)
            n274 = Increment(x=w319) -> (x+1=w317:i32)
            n275 = call "Get Channel Status.vi"("Channel"=w316, "Slave"=w317, "error in (no error)"=w321, "VISA resource name"=w320) -> ("error out"=w322:errorcluster, "Channel Enabled"=w315:bool)  [unwired: 5 in, 1 out]
            n276 = local read "Slaves ref array"() -> (w318:refnum<vi>[][])
            n277 = call "SubVI Set FP Channel-Guard value.vi"("Value"=w315, "Ch ID"=w316, "Slave ID"=w317, "Slaves ref array"=w318) -> ()  [unwired: 7 in, 1 out]
          }
        }
        n278 = Enqueue Element(queue=w289, element="slaves update", error in (no error)=w288) -> (error out=w287:errorcluster)  [unwired: 1 in, 2 out]
        n279 = local read "FP"() -> (w302:refnum<vi>[])
        n280 = call "SubVI Set Front panel elements.vi"("error in (passthrough)"=w287, "Array"=w302) -> ("error out"=w303:errorcluster)  [unwired: 9 in]
        n281 = local write "error"(w303) -> ()
      }
      event "Get Status": Value Change {
        n282 = event-data() -> ()  [unwired: 1 in, 6 out]
        n283 = local read "FP"() -> (w341:refnum<vi>[])
        n284 = call "SubVI Set Front panel elements.vi"("Enable elements (T)"=FALSE, "Array"=w341) -> ("error out"=w336:errorcluster)  [unwired: 9 in]
        n285 = local read "VISA"() -> (w337:refnum<visa-resource-name>)
        n286 = call "Get MX Status.vi"("error in (no error)"=w336, "VISA resource name"=w337) -> ("error out"=w335:errorcluster, "Ready?"=→"Ready?":bool, "Enabled"=→"Enabled":bool, "TRG Polarity Positive"=w330:bool, "Local?"=w334:bool, "TRG External"=w326:bool)  [unwired: 3 in, 1 out]
        n287 = local read "FP"() -> (w342:refnum<vi>[])
        n288 = Select(t=enum32{"Remote", "Local"}."Local" ("Operation"), s=w334, f=enum32{"Remote", "Local"}."Remote" ("Operation")) -> (s? t:f=w331:enum32{"Remote", "Local"})
        n289 = Select(t=enum32{"Positive", "Negative"}."Positive" ("Trigger polarity"), s=w330, f=enum32{"Positive", "Negative"}."Negative" ("Trigger polarity")) -> (s? t:f=w327:enum32{"Positive", "Negative"})
        n290 = Select(t=enum32{"Internal", "External"}."External" ("Trigger source"), s=w326, f=enum32{"Internal", "External"}."Internal" ("Trigger source")) -> (s? t:f=w323:enum32{"Internal", "External"})
        n291 = call "SubVI Set Front panel elements.vi"("error in (passthrough)"=w335, "Array"=w342) -> ("error out"=w343:errorcluster)  [unwired: 9 in]
        n292 = local write "Operation"(w331) -> ()
        n293 = local write "Trigger polarity"(w327) -> ()
        n294 = local write "Trigger source"(w323) -> ()
        n295 = local write "error"(w343) -> ()
      }
      event "no sequences get": Value Change {
        n296 = event-data() -> ()  [unwired: 1 in, 6 out]
        n297 = local read "FP"() -> (w349:refnum<vi>[])
        n298 = call "SubVI Set Front panel elements.vi"("Enable elements (T)"=FALSE, "Array"=w349) -> ("error out"=w347:errorcluster)  [unwired: 9 in]
        n299 = local read "VISA"() -> (w345:refnum<visa-resource-name>)
        n300 = call "Get Number of Sequences.vi"("error in (no error)"=w347, "VISA resource name"=w345) -> ("error out"=w346:errorcluster, "Number of sequences"=w344:i32)  [unwired: 7 in, 1 out]
        n301 = local read "FP"() -> (w350:refnum<vi>[])
        n302 = local write "Number of sequence lines:"(w344) -> ()
        n303 = call "SubVI Set Front panel elements.vi"("error in (passthrough)"=w346, "Array"=w350) -> ("error out"=w351:errorcluster)  [unwired: 9 in]
        n304 = local write "error"(w351) -> ()
      }
      event "sequence editor": Value Change {
        n305 = event-data() -> ()  [unwired: 1 in, 6 out]
        n306 = Enqueue Element(queue=w353, element="FP open") -> ()  [unwired: 2 in, 3 out]
      }
      event "Load sq to MX": Value Change {
        n307 = event-data() -> ()  [unwired: 1 in, 6 out]
        n308 = disable-structure shown="Default" {
          disable-tunnel: w358 -> [w390]
          disable-tunnel: [w375] -> w357
          disable-tunnel: [w374] -> w356
          frame Enabled {
            # "Get actual values from Sequence editor.vi"
            n309 = property class="VI"(reference=w390) -> ("Panel"=w389:refnum<vi>)  [unwired: 1 in, 2 out]
            n310 = property class="Pnl"(reference=w389) -> (reference out=w376:refnum<vi>, "Controls[]"=w377:refnum<vi>[])  [unwired: 1 in, 1 out]
            n311 = Close Reference(reference=w376) -> ()  [unwired: 1 in, 1 out]
            n312 = Close Reference(reference=w377) -> ()  [unwired: 1 in, 1 out]
            n313 = for {
              tunnel: w377 -> [w392] mode=indexing
              tunnel: [w391] -> w379 mode=indexing
              n314 = property class="Ctl"(reference=w392) -> ("Label.Text"=w391:string)  [unwired: 1 in, 2 out]
            }
            n315 = call "Search Unsorted 1D Array.vim"("element"="Sequence" ("Label.Text"), "unsorted 1D array"=w379) -> ("index of element"=w381:i32)  [unwired: 9 in]
            n316 = call "Search Unsorted 1D Array.vim"("element"="Timing\ndelay" ("Label.Text"), "unsorted 1D array"=w379) -> ("index of element"=w387:i32)  [unwired: 9 in]
            n317 = Index Array(array=w377, index=w381) -> (element=w382:refnum<vi>)
            n318 = property class="Ctl"(reference=w382) -> ("Value"=w383:variant)  [unwired: 1 in, 2 out]
            n319 = Index Array(array=w377, index=w387) -> (element=w386:refnum<vi>)
            n320 = property class="Ctl"(reference=w386) -> ("Value"=w385:variant)  [unwired: 1 in, 2 out]
            n321 = Variant To Data(type=u8[] [] ("Ch. bytes 2"), Variant=w385) -> (data=w374:u8[])  [unwired: 1 in, 1 out]
            n322 = Variant To Data(type=bool[][] [], Variant=w383) -> (data=w375:bool[][])  [unwired: 1 in, 1 out]
          }
        }
        n323 = Array Size(array=w356) -> (size(s)=w355:i32)
        n324 = Equal To 0?(x=w355) -> (x = 0?=w354:bool)
        n325 = case shown="False" w354 {
          tunnel: w357 -> [w364 _]
          tunnel: w356 -> [w363 _]
          frame False {
            n326 = local read "FP"() -> (w368:refnum<vi>[])
            n327 = call "Sequences to Bytes.vi"("Channel states"=w364) -> ("Ch. bytes 2"=w371:u8[], "Ch. bytes 1"=w372:u8[])  [unwired: 9 in]
            n328 = call "SubVI Set Front panel elements.vi"("Enable elements (T)"=FALSE, "Array"=w368) -> ("error out"=w366:errorcluster)  [unwired: 9 in]
            n329 = local read "VISA"() -> (w365:refnum<visa-resource-name>)
            n330 = call "Load Sequences.vi"("Byte 2 Ch."=w371, "Byte 3 Timing Delay"=w363, "Byte 1 Ch."=w372, "error in (no error)"=w366, "VISA resource name"=w365) -> ("error out"=w361:errorcluster, "VISA resource name out"=w359:refnum<visa-resource-name>)  [unwired: 5 in]
            n331 = local read "FP"() -> (w369:refnum<vi>[])
            n332 = call "Get Number of Sequences.vi"("error in (no error)"=w361, "VISA resource name"=w359) -> ("error out"=w360:errorcluster, "Number of sequences"=w362:i32)  [unwired: 7 in, 1 out]
            n333 = call "SubVI Set Front panel elements.vi"("error in (passthrough)"=w360, "Array"=w369) -> ("error out"=w370:errorcluster)  [unwired: 9 in]
            n334 = local write "error"(w370) -> ()
            n335 = local write "Number of sequence lines:"(w362) -> ()
          }
          frame True {
            n336 = One Button Dialog(message="Sequence matrix is empty.\nUse sequence editor to create\nsequence or load sequence\nfrom file.") -> ()  [unwired: 1 in, 1 out]
          }
        }
      }
      event "set sq line": Value Change {
        n337 = event-data() -> ()  [unwired: 1 in, 6 out]
        n338 = disable-structure shown="Default" {
          disable-tunnel: w406 -> [w417]
          disable-tunnel: [w407] -> w401
          frame Enabled {
            # "Get actual values from Sequence editor.vi"
            n339 = property class="VI"(reference=w417) -> ("Panel"=w416:refnum<vi>)  [unwired: 1 in, 2 out]
            n340 = property class="Pnl"(reference=w416) -> (reference out=w408:refnum<vi>, "Controls[]"=w409:refnum<vi>[])  [unwired: 1 in, 1 out]
            n341 = Close Reference(reference=w408) -> ()  [unwired: 1 in, 1 out]
            n342 = Close Reference(reference=w409) -> ()  [unwired: 1 in, 1 out]
            n343 = for {
              tunnel: w409 -> [w419] mode=indexing
              tunnel: [w418] -> w411 mode=indexing
              n344 = property class="Ctl"(reference=w419) -> ("Label.Text"=w418:string)  [unwired: 1 in, 2 out]
            }
            n345 = call "Search Unsorted 1D Array.vim"("element"="Sequence" ("Label.Text"), "unsorted 1D array"=w411) -> ("index of element"=w413:i32)  [unwired: 9 in]
            n346 = Index Array(array=w409, index=w413) -> (element=w414:refnum<vi>)
            n347 = property class="Ctl"(reference=w414) -> ("Value"=w415:variant)  [unwired: 1 in, 2 out]
            n348 = Variant To Data(type=bool[][] [], Variant=w415) -> (data=w407:bool[][])  [unwired: 1 in, 1 out]
          }
        }
        n349 = Decrement(x="Set to sequence line:") -> (x-1=w393:i32)
        n350 = local read "FP"() -> (w404:refnum<vi>[])
        n351 = Index Array(array=w401, index (row)=w393) -> (element=w400:bool[])  [unwired: 1 in]
        n352 = call "SubVI Set Front panel elements.vi"("Enable elements (T)"=FALSE, "Array"=w404) -> ("error out"=w402:errorcluster)  [unwired: 9 in]
        n353 = local read "VISA"() -> (w399:refnum<visa-resource-name>)
        n354 = call "Set Sequence Line.vi"("error in (no error)"=w402, "Sequence Line"=w400, "VISA resource name"=w399) -> ("error out"=w398:errorcluster)  [unwired: 7 in, 1 out]
        n355 = local read "FP"() -> (w405:refnum<vi>[])
        n356 = call "SubVI Set Front panel elements.vi"("error in (passthrough)"=w398, "Array"=w405) -> ("error out"=w397:errorcluster)  [unwired: 9 in]
        n357 = property on="dummy for event \"check channels\"" class="Bool (strict)"(error in=w397, "Val(Sgnl)"=TRUE) -> (error out=w396:errorcluster)  [unwired: 1 in, 1 out]
        n358 = local write "error"(w396) -> ()
      }
      event "Get sq from MX": Value Change {
        n359 = event-data() -> ()  [unwired: 1 in, 6 out]
        n360 = local read "FP"() -> (w421:refnum<vi>[])
        n361 = call "SubVI Set Front panel elements.vi"("Enable elements (T)"=FALSE, "Array"=w421) -> ("error out"=w439:errorcluster)  [unwired: 9 in]
        n362 = local read "VISA"() -> (w437:refnum<visa-resource-name>)
        n363 = call "Get Sequences.vi"("error in (no error)"=w439, "VISA resource name"=w437) -> ("error out"=w438:errorcluster, "Byte 3 Delay"=w431:u8[], "Byte 2 Ch."=w434:u8[], "Byte 1 Ch."=w435:u8[])  [unwired: 5 in, 1 out]
        n364 = Array Size(array=w431) -> (size(s)=w436:i32)
        n365 = local read "FP"() -> (w440:refnum<vi>[])
        n366 = call "Bytes to Sequences.vi"("Ch. bytes 2"=w434, "Ch. bytes 1"=w435) -> ("Array"=w432:bool[][])  [unwired: 9 in]
        n367 = call "SubVI Set Front panel elements.vi"("error in (passthrough)"=w438, "Array"=w440) -> ("error out"=w441:errorcluster)  [unwired: 9 in]
        n368 = local write "Number of sequence lines:"(w436) -> ()
        n369 = local write "error"(w441) -> ()
        n370 = disable-structure shown="Default" {
          disable-tunnel: w433 -> [w455]
          disable-tunnel: w432 -> [w444]
          disable-tunnel: w431 -> [w443]
          disable-tunnel: w430 -> [w442]
          disable-tunnel: [w442] -> w422
          frame Enabled {
            # "Push actual values to Sequence editor.vi"
            n371 = property class="VI"(reference=w455) -> ("Panel"=w454:refnum<vi>)  [unwired: 1 in, 2 out]
            n372 = property class="Pnl"(reference=w454) -> (reference out=w445:refnum<vi>, "Controls[]"=w446:refnum<vi>[])  [unwired: 1 in, 1 out]
            n373 = Close Reference(reference=w445) -> ()  [unwired: 1 in, 1 out]
            n374 = Close Reference(reference=w446) -> ()  [unwired: 1 in, 1 out]
            n375 = for {
              tunnel: w446 -> [w457] mode=indexing
              tunnel: [w456] -> w447 mode=indexing
              n376 = property class="Ctl"(reference=w457) -> ("Label.Text"=w456:string)  [unwired: 1 in, 2 out]
            }
            n377 = call "Search Unsorted 1D Array.vim"("element"="Sequence" ("Label.Text"), "unsorted 1D array"=w447) -> ("index of element"=w449:i32)  [unwired: 9 in]
            n378 = call "Search Unsorted 1D Array.vim"("element"="Timing\ndelay" ("Label.Text"), "unsorted 1D array"=w447) -> ("index of element"=w452:i32)  [unwired: 9 in]
            n379 = Index Array(array=w446, index=w449) -> (element=w450:refnum<vi>)
            n380 = property class="Ctl"(reference=w450, "Value"=w444) -> ()  [unwired: 1 in, 2 out]
            n381 = Index Array(array=w446, index=w452) -> (element=w451:refnum<vi>)
            n382 = property class="Ctl"(reference=w451, "Value"=w443) -> ()  [unwired: 1 in, 2 out]
          }
        }
        n383 = Enqueue Element(queue=w422, element="sequence fill missing collumns") -> (queue out=w426:refnum<queue>, error out=w429:errorcluster)  [unwired: 2 in, 1 out]
        n384 = Enqueue Element(queue=w426, element="index timing update", error in (no error)=w429) -> (queue out=w427:refnum<queue>, error out=w428:errorcluster)  [unwired: 1 in, 1 out]
        n385 = Enqueue Element(queue=w427, element="scrollbar sync", error in (no error)=w428) -> ()  [unwired: 1 in, 3 out]
      }
    }
  }
  n386 = flat-sequence {
    tunnel: w3 -> [w459]
    tunnel: w7 -> [w460]
    tunnel: w16 -> [w461]
    tunnel: [w461] -> w6
    tunnel: [w460] -> w5
    tunnel: [w458] -> w4
    tunnel: w6 -> [_]
    tunnel: w5 -> [w466]
    tunnel: w4 -> [w463]
    frame #0 {
      n387 = Close Reference(reference=w459) -> (error out=w458:errorcluster)  [unwired: 1 in]
    }
    frame #1 {
      n388 = local read "VISA"() -> (w468:refnum<visa-resource-name>)
      n389 = Enqueue Element(queue=w466, element="quit") -> (error out=w464:errorcluster)  [unwired: 2 in, 2 out]
      n390 = call "Close.vi"("VISA resource name"=w468) -> ("error out"=w467:errorcluster)  [unwired: 10 in]
      n391 = Merge Errors(w467, w464, w463) -> (w462:errorcluster)
      "error" <- w462
      n392 = disable-structure shown="Default" {
        disable-tunnel: w462 -> [_ _]
        frame condition #0 (active) {
          n393 = Stop(stop? (T)=TRUE) -> ()
        }
        frame condition #1 {
          n394 = Quit LabVIEW(quit? (T)=TRUE) -> ()
        }
      }
    }
  }
